vi "DCC_LoadFromLVSET.vi"(8 "Error In":errorcluster) -> (0 "Error Out":errorcluster, 5 "Array":T1[](array[typedef]) {"Cooler Volt [V]" scale=0.0..5.0; "Cooler Current [A]" scale=0.0..2.0; "Connector 3"."Gain/HV [%]" scale=0.0..100.0; "Connector 1"."Gain/HV [%]" scale=0.0..100.0})   [LabVIEW 2019]
doc: "The \"Load from LVSET.vi\" loads the *.lvset file specified by the user and translate it into the correct DCC control cluster values.\n\nMarch 2019\nFrank Quadt & Stefan Smietana\ninfo@becker-hickl.com"
uses:
  DCC_Controls/DCC_ControlCluster.ctl
  DCC_Controls/DCC_Connector1.ctl
  DCC_Controls/DCC_Connector2.ctl
panel:
  # "(c) 2018 Becker & Hickl GmbH\n     ALL RIGHTS RESERVED."
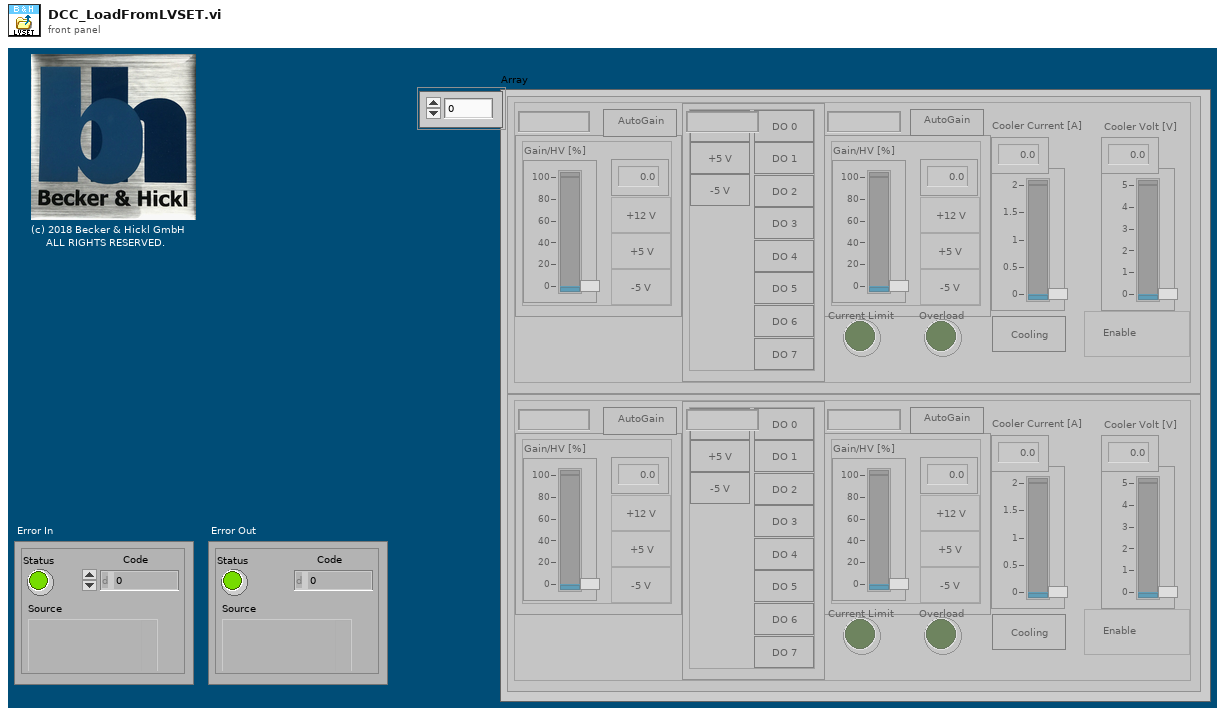
[diagram p1: front panel]
types:
  T1 = typedef "DCC_ControlCluster.ctl" = cluster{"Connector 1":T2, "Connector 2":T3, "Connector 3":T2, "Cooler Current [A]":dbl, "Cooler Volt [V]":dbl, "Cooling":bool, "Enable Outputs":bool, "AutoGain1":bool, "AutoGain3":bool, "Current Limit":bool, "Overload":bool, "LabelCon1":string, "LabelCon2":string, "LabelCon3":string}
  T2 = typedef "DCC_Connector1.ctl" = cluster{"Gain/HV [%]":dbl, "+12V":bool, "+5V":bool, "-5V":bool}
  T3 = typedef "DCC_Connector2.ctl" = cluster{"+12V":bool, "+5V":bool, "-5V":bool, "DO0":bool, "DO1":bool, "DO2":bool, "DO3":bool, "DO4":bool, "DO5":bool, "DO6":bool, "DO7":bool}
  T4 = enum16{"open", "replace", "create", "open or create", "replace or create", "replace or create with confirmation"}
  T5 = enum16{"big-endian, network order", "native, host order", "little-endian"}
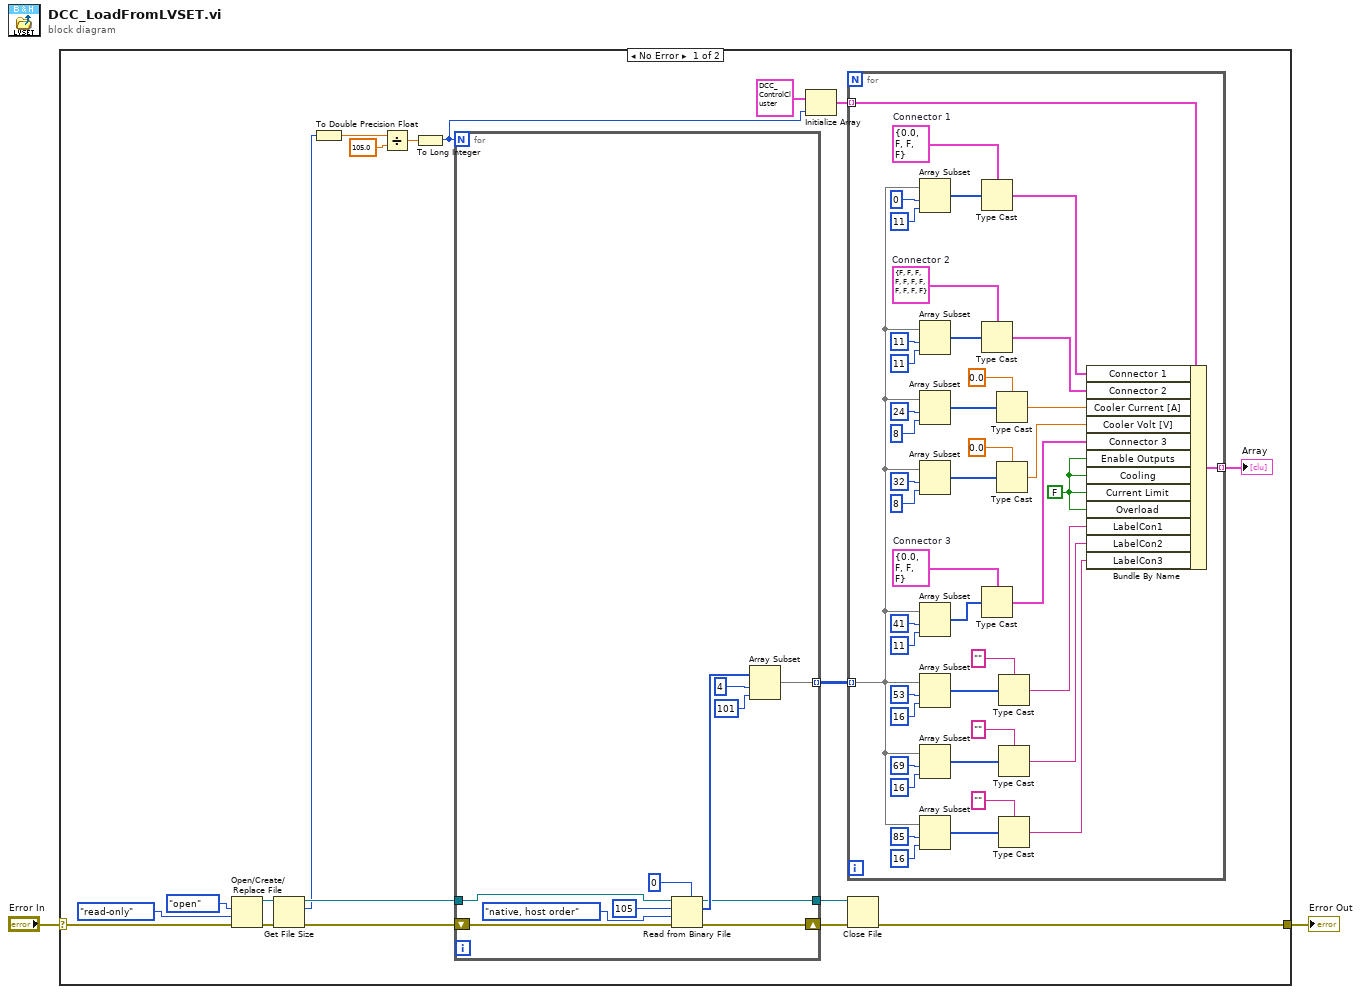
[diagram p0: block diagram]
diagram:
  n1 = case shown="No Error" "Error In" {
    selector: "Error In" -> [w21 w77]
    tunnel: [w20 w77] -> w1
    frame No Error {
      n2 = Open/Create/Replace File(error in=w21, operation (0:open)=T4."open", access (0:read/write)=enum16{"read/write", "read-only", "write-only"}."read-only") -> (refnum out=w14:refnum<file>, error out=w12:errorcluster)  [unwired: 3 in, 1 out]
      n3 = Get File Size(file=w14, error in=w12) -> (refnum out=w13:refnum<file>, size (in bytes)=w9:i64, 0:w11:errorcluster)
      n4 = To Double Precision Float(number=w9) -> (double precision float=w8:dbl)
      n5 = Divide(x=w8, y=105.0) -> (x/y=w7:dbl)
      n6 = To Long Integer(number=w7) -> (32bit integer=w3:i32)
      n7 = for {
        N: w3 -> [_]
        tunnel: w13 -> [w29]
        tunnel: [w26] -> w17
        shift-right: [w25] -> w16
        shift-left: w11 -> [w30]
        tunnel: [w22] -> w15 mode=indexing
        n8 = Read from Binary File(5:u8 0 ("Numeric"), 8:w30, 9:T5."native, host order" ("byte order (0:big-endian, network order)"), 10:105, 11:w29) -> (0:w25:errorcluster, 2:w27:u8[], 3:w26:refnum<file>)  [unwired: 1 in, 1 out]
        n9 = Array Subset(array=w27, index=4, length=101) -> (w22:u8[])
      }
      n10 = Initialize Array(T1 {"Connector 1"={"Gain/HV [%]"=0.0, "+12V"=FALSE, "+5V"=FALSE, "-5V"=FALSE}, "Connector 2"={"+12V"=FALSE, "+5V"=FALSE, "-5V"=FALSE, "DO0"=FALSE, "DO1"=FALSE, "DO2"=FALSE, "DO3"=FALSE, "DO4"=FALSE, "DO5"=FALSE, "DO6"=FALSE, "DO7"=FALSE}, "Connector 3"={"Gain/HV [%]"=0.0, "+12V"=FALSE, "+5V"=FALSE, "-5V"=FALSE}, "Cooler Current [A]"=0.0, "Cooler Volt [V]"=0.0, "Cooling"=FALSE, "Enable Outputs"=FALSE, "AutoGain1"=FALSE, "AutoGain3"=FALSE, "Current Limit"=FALSE, "Overload"=FALSE, "LabelCon1"="Connector 1", "LabelCon2"="Connector 2", "LabelCon3"="Connector 3"} ("Module"), w3) -> (w5:T1[])
      n11 = for {
        tunnel: w5 -> [w75] mode=indexing
        tunnel: [w76] -> w4 mode=indexing
        tunnel: w15 -> [w37] mode=indexing
        w64 = T3 {"+12V"=FALSE, "+5V"=FALSE, "-5V"=FALSE, "DO0"=FALSE, "DO1"=FALSE, "DO2"=FALSE, "DO3"=FALSE, "DO4"=FALSE, "DO5"=FALSE, "DO6"=FALSE, "DO7"=FALSE}  # Connector 2
        w51 = T2 {"Gain/HV [%]"=0.0, "+12V"=FALSE, "+5V"=FALSE, "-5V"=FALSE}  # Connector 3
        w71 = T2 {"Gain/HV [%]"=0.0, "+12V"=FALSE, "+5V"=FALSE, "-5V"=FALSE}  # Connector 1
        w36 = FALSE
        n12 = Array Subset(array=w37, index=0, length=11) -> (w72:u8[])
        n13 = Array Subset(array=w37, index=11, length=11) -> (w65:u8[])
        n14 = Array Subset(array=w37, index=24, length=8) -> (w59:u8[])
        n15 = Array Subset(array=w37, index=32, length=8) -> (w55:u8[])
        n16 = Array Subset(array=w37, index=41, length=11) -> (w52:u8[])
        n17 = Array Subset(array=w37, index=53, length=16) -> (w47:u8[])
        n18 = Array Subset(array=w37, index=69, length=16) -> (w44:u8[])
        n19 = Array Subset(array=w37, index=85, length=16) -> (w39:u8[])
        n20 = Type Cast(type=w71, x=w72) -> (*(type *) &x=w70:T2)
        n21 = Type Cast(type=w64, x=w65) -> (*(type *) &x=w63:T3)
        n22 = Type Cast(type=w51, x=w52) -> (*(type *) &x=w50:T2)
        n23 = Type Cast(type=0.0, x=w59) -> (*(type *) &x=w58:dbl)
        n24 = Type Cast(type=0.0, x=w55) -> (*(type *) &x=w54:dbl)
        n25 = Type Cast(type="", x=w47) -> (*(type *) &x=w35:string)
        n26 = Type Cast(type="", x=w44) -> (*(type *) &x=w34:string)
        n27 = Type Cast(type="", x=w39) -> (*(type *) &x=w33:string)
        n28 = Bundle By Name(cluster=w75, "Connector 1"=w70, "Connector 2"=w63, "Cooler Current [A]"=w58, "Cooler Volt [V]"=w54, "Connector 3"=w50, "Enable Outputs"=w36, "Cooling"=w36, "Current Limit"=w36, "Overload"=w36, "LabelCon1"=w35, "LabelCon2"=w34, "LabelCon3"=w33) -> (w76:T1)
      }
      "Array" <- w4
      n29 = Close File(refnum=w17, error in=w16) -> (error out=w20:errorcluster)  [unwired: 1 out]
    }
    frame Error {
    }
  }
  "Error Out" <- w1
